vi "Initiate.vi"(8 "error in (no error)":errorcluster, 11 "VISA resource name":refnum<visa-resource-name>) -> (0 "error out":errorcluster, 3 "VISA resource name out":refnum<visa-resource-name>)   [LabVIEW 2014, in "Agilent ESA PSA Series.lvlib"]
doc: "Initiates a trace sweep. After you call this VI, the instrument leaves the idle state and waits for a trigger.\n\n<B>Note:</B>\n\nUse this VI only with other low-level VIs. The high-level VIs automatically incorporate this functionality. This VI does not check the instrument status."
uses:
  Agilent ESA PSA Series.lvlib
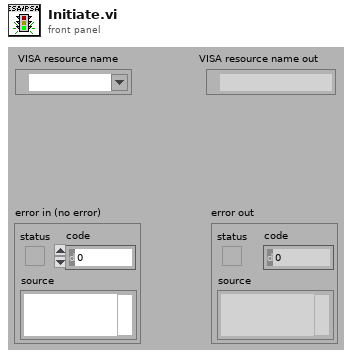
[diagram p1: front panel]
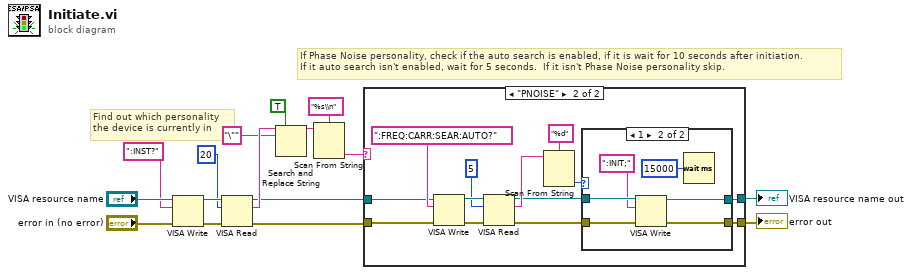
[diagram p0: block diagram]
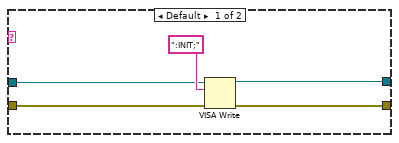
[diagram p2: hidden frame]
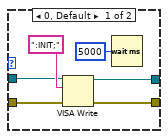
[diagram p3: hidden frame]
diagram:
  # "If Phase Noise personality, check if the auto search is enabled, if it is wait for 10 seconds after initiation.\nIf it auto search isn't enabled, wait for 5 seconds.  If it isn't Phase Noise personality skip."
  # "Find out which personality\nthe device is currently in"
  n1 = VISA Write(VISA resource name="VISA resource name", write buffer=":INST?", error in (no error)="error in (no error)") -> (VISA resource name out=w12:refnum<visa-resource-name>, error out=w13:errorcluster)  [unwired: 1 out]
  n2 = VISA Read(VISA resource name=w12, byte count=u32 20, error in (no error)=w13) -> (VISA resource name out=w4:refnum<visa-resource-name>, read buffer=w10:string, error out=w3:errorcluster)  [unwired: 1 out]
  n3 = Search and Replace String(replace all?=TRUE ("replace all? (F)"), input string=w10, search string="\"") -> (result string=w7:string)  [unwired: 5 in, 3 out]
  n4 = Scan From String(format string="%s\\n", input string=w7) -> (output 1=w5:string)  [unwired: 3 in, 3 out]
  n5 = case shown="\"PNOISE\"" w5 {
    tunnel: w4 -> [w20 w33]
    tunnel: w3 -> [w19 w32]
    tunnel: [w18 w23] -> w2
    tunnel: [w17 w22] -> w1
    frame Default {
      n6 = VISA Write(VISA resource name=w20, write buffer=":INIT;", error in (no error)=w19) -> (VISA resource name out=w18:refnum<visa-resource-name>, error out=w17:errorcluster)  [unwired: 1 out]
    }
    frame "PNOISE" {
      n7 = VISA Write(VISA resource name=w33, write buffer=":FREQ:CARR:SEAR:AUTO?", error in (no error)=w32) -> (VISA resource name out=w30:refnum<visa-resource-name>, error out=w31:errorcluster)  [unwired: 1 out]
      n8 = VISA Read(VISA resource name=w30, byte count=u32 5, error in (no error)=w31) -> (VISA resource name out=w25:refnum<visa-resource-name>, read buffer=w28:string, error out=w24:errorcluster)  [unwired: 1 out]
      n9 = Scan From String(format string="%d", input string=w28) -> (output 1=w26:i32)  [unwired: 3 in, 3 out]
      n10 = case shown="1" w26 {
        tunnel: w25 -> [w39 w45]
        tunnel: w24 -> [w38 w44]
        tunnel: [w36 w42] -> w23
        tunnel: [w37 w41] -> w22
        frame 0, Default {
          n11 = VISA Write(VISA resource name=w39, write buffer=":INIT;", error in (no error)=w38) -> (VISA resource name out=w36:refnum<visa-resource-name>, error out=w37:errorcluster)  [unwired: 1 out]
          n12 = Wait (ms)(milliseconds to wait=u32 5000) -> ()  [unwired: 1 out]
        }
        frame 1 {
          n13 = VISA Write(VISA resource name=w45, write buffer=":INIT;", error in (no error)=w44) -> (VISA resource name out=w42:refnum<visa-resource-name>, error out=w41:errorcluster)  [unwired: 1 out]
          n14 = Wait (ms)(milliseconds to wait=u32 15000) -> ()  [unwired: 1 out]
        }
      }
    }
  }
  "error out" <- w1
  "VISA resource name out" <- w2
